vi "Motion Status.vi"(8 "error in (no error)":errorcluster, 9 "Axis (1..4)":T1=3 items=["X"=1, "Y"=2, "Z"=3, "T"=4], 11 "VXMx2 in":refnum<class "VXMx2.lvclass">) -> (0 "error out":errorcluster, 1 "Motion Stopped":bool, 3 "VXMx2 out":refnum<class "VXMx2.lvclass">, 4 "Limit Switch Activated":bool)   [LabVIEW 2019, in "VXMx2.lvclass"]
doc: "This VI is for reading motion controller status during motion"
uses:
  VXMx2.lvclass
  <instrlib>/Velmex VXM/Public/VXM Axis.ctl
  VXMx2.lvclass/VXMx2.ctl
  Support/MessageAPI/UIMessage.ctl
  SendMessage/SendMessage.lvclass
  <instrlib>/Velmex VXM/Velmex VXM.lvlib
panel:
  out "X, Y Positions, eng units":dbl[](array[numeric])
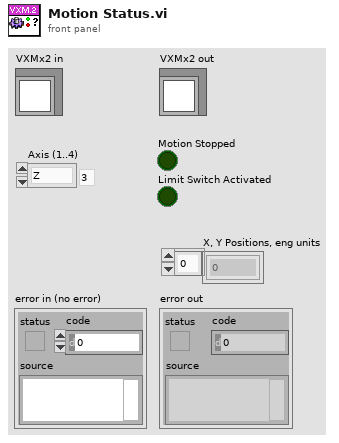
[diagram p1: front panel]
types:
  T1 = typedef "Velmex VXM.lvlib/VXM Axis.ctl" = u16
  T2 = typedef "UIMessage.ctl" = cluster{"EventCode":i32, "Numeric":dbl, "String":string, "Variant":variant}
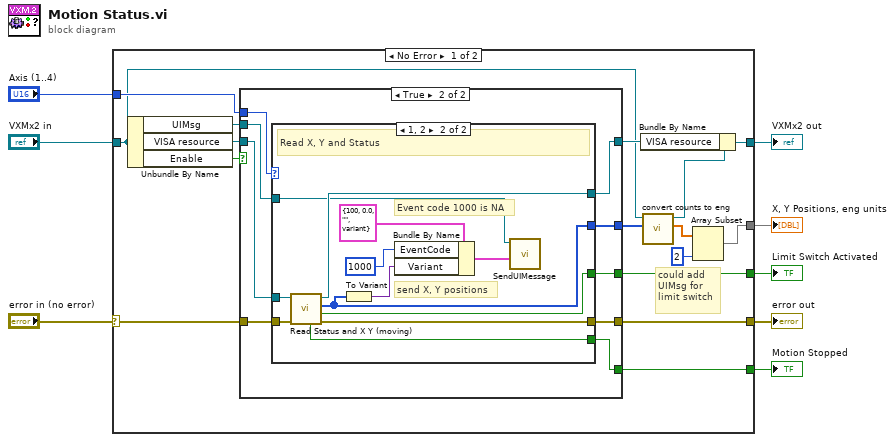
[diagram p0: block diagram]
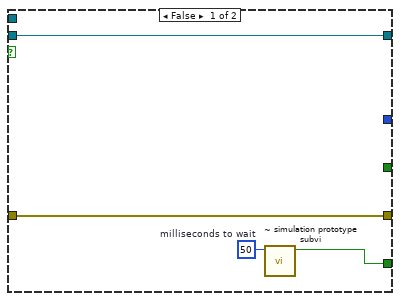
[diagram p2: hidden frame]
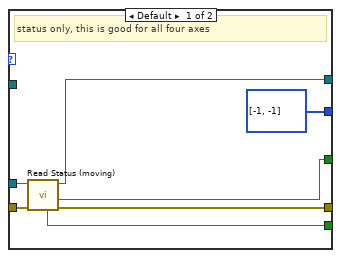
[diagram p3: hidden frame]
diagram:
  n1 = case shown="No Error" "error in (no error)" {
    selector: "error in (no error)" -> [w21 w58]
    tunnel: [w20 w58] -> w7
    tunnel: [w19 w57] -> w5
    tunnel: "VXMx2 in" -> [w13 w57]
    tunnel: [w24 _] -> w4
    tunnel: [w17 _] -> w3
    tunnel: "Axis (1..4)" -> [w22 _]
    tunnel: [w10 _] -> w1
    frame No Error {
      # "could add \nUIMsg for \nlimit switch"
      n2 = Unbundle By Name(w13) -> ("UIMsg"=w16:refnum<class "SendMessage.lvclass">, "VISA resource"=w23:refnum<visa-resource-name>, "Enable"=w15:bool)
      n3 = case shown="True" w15 {
        tunnel: [_ w37] -> w24
        tunnel: w23 -> [w28 w36]
        tunnel: w22 -> [_ w35]
        tunnel: w21 -> [w27 w34]
        tunnel: [w27 w33] -> w20
        tunnel: [w28 w32] -> w18
        tunnel: [_ w31] -> w14
        tunnel: [w26 w30] -> w17
        tunnel: w16 -> [_ w29]
        frame False {
          w25 = u32 50  # milliseconds to wait
          n4 = call "~ simulation prototype subvi.vi"("milliseconds to wait"=w25) -> ("Motion Stopped = T"=w26:bool)  [unwired: 10 in]
        }
        frame True {
          n5 = case shown="1, 2" w35 {
            tunnel: w34 -> [w44 w56]
            tunnel: [w43 w55] -> w33
            tunnel: [w40 w51] -> w30
            tunnel: w36 -> [w42 w54]
            tunnel: [w38 w53] -> w32
            tunnel: [w41 w52] -> w37
            tunnel: [i32[] [-1, -1] ("Positions, counts") w47] -> w31
            tunnel: w29 -> [_ w45]
            frame Default {
              # "status only, this is good for all four axes"
              n6 = call <instrlib>:"Read Status (moving).vi"("error in (no error)"=w44, "VISA resource name"=w42) -> ("error out"=w43:errorcluster, "Limit Switch Activated"=w41:bool, "VISA resource out"=w38:refnum<visa-resource-name>, "Motion Stopped"=w40:bool)  [unwired: 5 in, 1 out]
            }
            frame 1, 2 {
              # "Event code 1000 is NA"
              # "send X, Y positions"
              # "Read X, Y and Status"
              n7 = call <instrlib>:"Read Status and X Y (moving).vi"("error in (no error)"=w56, "VISA resource name"=w54) -> ("error out"=w55:errorcluster, "Limit Switch Activated"=w52:bool, "Positions, counts"=w47:i32[], "VISA resource out"=w53:refnum<visa-resource-name>, "Motion Stopped"=w51:bool)  [unwired: 4 in, 1 out]
              n8 = To Variant(anything=w47) -> (Variant=w48:variant)
              n9 = Bundle By Name(cluster=T2 {"EventCode"=100, "Numeric"=0.0, "String"="", "Variant"=variant} ("UIMsg"), "EventCode"=1000, "Variant"=w48) -> (w50:T2)
              n10 = call-dynamic "SendUIMessage.vi"("UIMsg"=w50, "SendMessage in"=w45) -> ()  [unwired: 8 in, 2 out]
            }
          }
        }
      }
      n11 = call "convert counts to eng.vi"("All Positions, counts"=w14, "VXMx2 in"=w13) -> ("All Positions, eng units"=w12:dbl[], "VXMx2 out"=w9:refnum<class "VXMx2.lvclass">)  [unwired: 6 in, 2 out]
      n12 = Bundle By Name(cluster=w9, "VISA resource"=w18) -> (w19:refnum<class "VXMx2.lvclass">)
      n13 = Array Subset(array=w12, length=2) -> (w10:dbl[])  [unwired: 1 in]
    }
    frame Error {
    }
  }
  "error out" <- w7
  "VXMx2 out" <- w5
  "Motion Stopped" <- w3
  "Limit Switch Activated" <- w4
  "X, Y Positions, eng units" <- w1
